vi "from_nodes.vi"(5 "edge type":refnum<class "Edge.lvclass">, 9 "node-b":refnum<class "Node.lvclass">, 10 "node-a":refnum<class "Node.lvclass">) -> (3 "new edge":refnum<class "Edge.lvclass">)   [LabVIEW 2020, in "graph.lvlib" / "Edge.lvclass"]
uses:
  Edge.lvclass
  Node/Node.lvclass
  Edge.lvclass/Edge.ctl
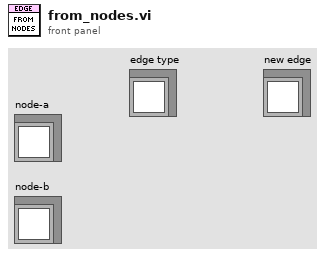
[diagram p1: front panel]
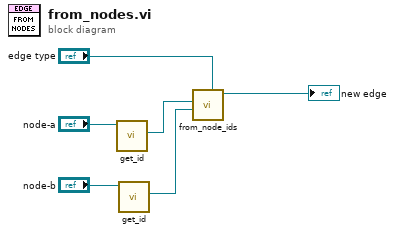
[diagram p0: block diagram]
diagram:
  n1 = call "get_id.vi"("node"="node-a") -> ("node-id"=w4:refnum<class "ID.lvclass">)  [unwired: 10 in]
  n2 = call "get_id.vi"("node"="node-b") -> ("node-id"=w3:refnum<class "ID.lvclass">)  [unwired: 10 in]
  n3 = call-dynamic "from_node_ids.vi"("edge type"="edge type", "sink-id"=w3, "source-id"=w4) -> ("new edge"=→"new edge":refnum<class "Edge.lvclass">)  [unwired: 8 in]
